vi "calc_prefix.vi"(10 "unit":string, 11 "Numeric in":dbl) -> (2 "prefix":string, 3 "Numeric out":dbl)   [LabVIEW 2025]
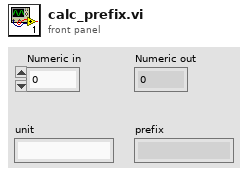
[diagram p1: front panel]
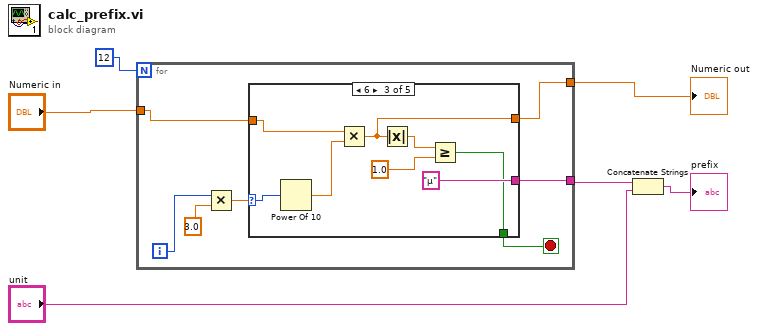
[diagram p0: block diagram]
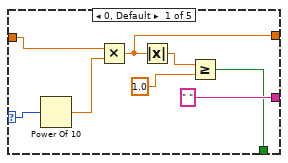
[diagram p2: hidden frame]
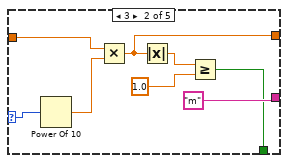
[diagram p3: hidden frame]
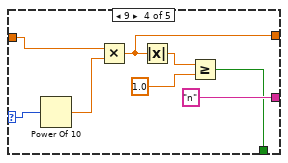
[diagram p4: hidden frame]
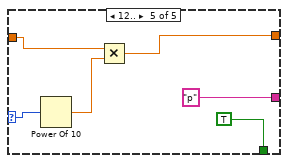
[diagram p5: hidden frame]
diagram:
  n1 = for {
    N: 12 -> [_]
    tunnel: "Numeric in" -> [w11]
    tunnel: [w12] -> w2
    tunnel: [w10] -> w6
    i -> [w7]
    stop <- w13 stop-if-true
    n2 = Multiply(x=w7, y=3.0) -> (x*y=w9:dbl)
    n3 = case shown="6" w9 {
      selector: w9 -> [w17 w23 w32 w41 w47]
      tunnel: [w15 w28 w30 w38 TRUE] -> w13
      tunnel: [" " "m" "µ" "n" "p"] -> w12
      tunnel: w11 -> [w16 w25 w31 w40 w46]
      tunnel: [w14 w22 w33 w39 w48] -> w10
      frame 0, Default {
        n4 = Power Of 10(x=w17) -> (10^x=w20:dbl)
        n5 = Multiply(x=w16, y=w20) -> (x*y=w14:dbl)
        n6 = Absolute Value(x=w14) -> (abs(x)=w19:dbl)
        n7 = Greater Or Equal?(x=w19, y=1.0) -> (x >= y?=w15:bool)
      }
      frame 3 {
        n8 = Power Of 10(x=w23) -> (10^x=w24:dbl)
        n9 = Multiply(x=w25, y=w24) -> (x*y=w22:dbl)
        n10 = Absolute Value(x=w22) -> (abs(x)=w27:dbl)
        n11 = Greater Or Equal?(x=w27, y=1.0) -> (x >= y?=w28:bool)
      }
      frame 6 {
        n12 = Power Of 10(x=w32) -> (10^x=w34:dbl)
        n13 = Multiply(x=w31, y=w34) -> (x*y=w33:dbl)
        n14 = Absolute Value(x=w33) -> (abs(x)=w36:dbl)
        n15 = Greater Or Equal?(x=w36, y=1.0) -> (x >= y?=w30:bool)
      }
      frame 9 {
        n16 = Power Of 10(x=w41) -> (10^x=w42:dbl)
        n17 = Multiply(x=w40, y=w42) -> (x*y=w39:dbl)
        n18 = Absolute Value(x=w39) -> (abs(x)=w44:dbl)
        n19 = Greater Or Equal?(x=w44, y=1.0) -> (x >= y?=w38:bool)
      }
      frame 12.. {
        n20 = Power Of 10(x=w47) -> (10^x=w50:dbl)
        n21 = Multiply(x=w46, y=w50) -> (x*y=w48:dbl)
      }
    }
  }
  "Numeric out" <- w6
  n22 = Concatenate Strings(w2, "unit") -> (→"prefix":string)
